vi "dbl2json.vi"(2 "error in (no error)":errorcluster, 3 "Numeric":dbl) -> (0 "error out":errorcluster, 1 "JSON":string)   [LabVIEW 2011, in "JSON.lvlib"]
uses:
  JSON.lvlib
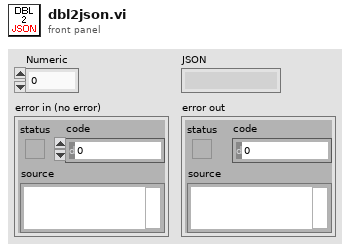
[diagram p1: front panel]
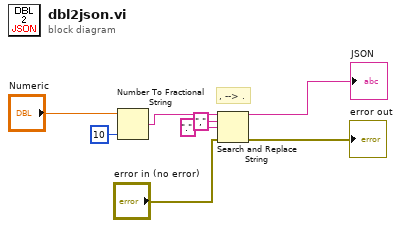
[diagram p0: block diagram]
diagram:
  # ", --> ."
  n1 = Number To Fractional String(number="Numeric", precision (6)=i16 10) -> (F-format string=w7:string)  [unwired: 2 in]
  n2 = Search and Replace String(input string=w7, search string=",", replace string="." ("replace string (\"\")"), error in="error in (no error)") -> (result string=→"JSON":string, error out=→"error out":errorcluster)  [unwired: 4 in, 2 out]
